vi "ex1_SimpleDAQ.vi"() -> ()   [LabVIEW 2010]
panel:
  in  "Acquire Start":bool
  out "CH2 Data":dbl[](graph)
  out "CH1 Data":dbl[](graph)
  in  "Acquire Stop":bool
  in  "Exit":bool
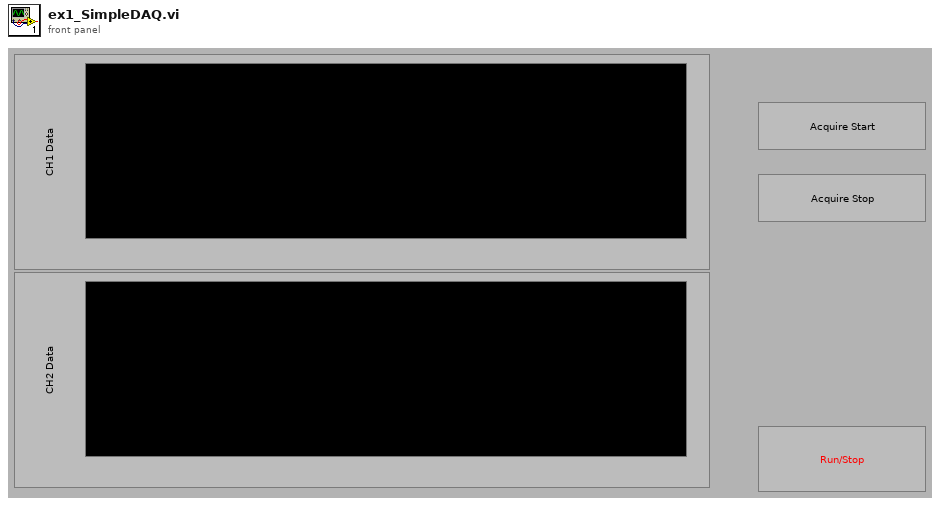
[diagram p1: front panel]
types:
  T1 = cluster{"Q_DblData":refnum<queue>, "DeviceHandle":u32, "Q_EventData":refnum<queue>, "Q_Int16Data":refnum<queue>}
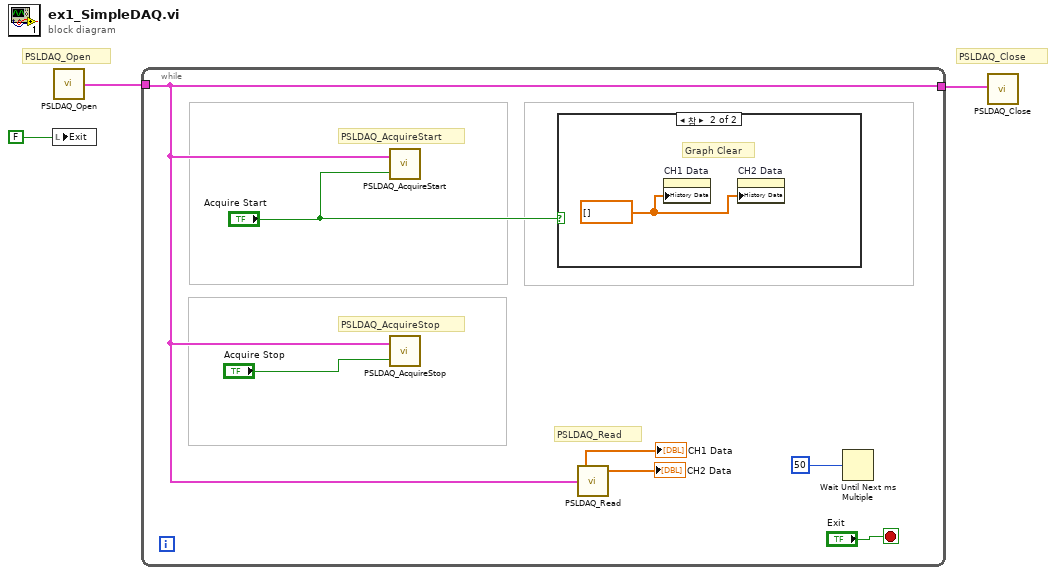
[diagram p0: block diagram]
diagram:
  # "PSLDAQ_Close"
  # "PSLDAQ_Open"
  n1 = local write "Exit"(FALSE ("Run Stop")) -> ()
  n2 = call "PSLDAQ_Open.vi"() -> ("Handle Out"=w2:T1)  [unwired: 1 in]
  n3 = while {
    tunnel: [w4] -> w1
    tunnel: w2 -> [w4]
    stop <- "Exit" stop-if-true
    # "PSLDAQ_Read"
    # "PSLDAQ_AcquireStop"
    # "PSLDAQ_AcquireStart"
    n4 = call "PSLDAQ_AcquireStart.vi"("Trigger"="Acquire Start", "Handle In"=w4) -> ()  [unwired: 1 in]
    n5 = call "PSLDAQ_AcquireStop.vi"("Trigger"="Acquire Stop", "Handle In"=w4) -> ()  [unwired: 1 in]
    n6 = case shown="참" "Acquire Start" {
      frame False {
      }
      frame True {
        w11 = dbl[] [] ("History Data")
        # "Graph Clear"
        n7 = property on="CH1 Data" class="WFChart (엄격한)"("History Data"=w11) -> ()  [unwired: 2 in, 2 out]
        n8 = property on="CH2 Data" class="WFChart (엄격한)"("History Data"=w11) -> ()  [unwired: 2 in, 2 out]
      }
    }
    n9 = call "PSLDAQ_Read.vi"("Handle In"=w4) -> ("CH2 Data"=→"CH2 Data":dbl[], "CH1 Data"=→"CH1 Data":dbl[])  [unwired: 3 out]
    n10 = Wait Until Next ms Multiple(millisecond multiple=u32 50) -> ()  [unwired: 1 out]
  }
  n11 = call "PSLDAQ_Close.vi"("Handle In"=w1) -> ()
